vi "Process.vi"(8 "error in":errorcluster, 11 "Inst.Krohn-Hite-7008":refnum<class "Inst.Krohn-Hite-7008.lvclass">) -> (0 "error out":errorcluster, 3 "Inst.Krohn-Hite-7008 out":refnum<class "Inst.Krohn-Hite-7008.lvclass">)   [LabVIEW 2019, in "Inst.KH7008.lvlib" / "Inst.Krohn-Hite-7008.lvclass"]
doc: "---------------------------------------------------------------\nJKI State Machine Objects™\nhttp://jki.net/state-machine-objects/\nCopyright (C) 2005-2015, JKI <info@jki.net>\nALL RIGHTS RESERVED"
uses:
  Inst.Krohn-Hite-7008.lvclass
  <userlib>/LevyLab/Instrument Framework/Instrument/Instrument.lvclass
  <userlib>/LevyLab/RemoteControl/RemoteControl/Typedefs/Message--Cluster.ctl
  <userlib>/LevyLab/RemoteControl/RemoteControl/RemoteControl.lvclass
  Typedefs/PrivateEvents--Inst.KH7008.MessageToProcess.ctl
  Typedefs/Inst.KH7008.Commands--Enum.ctl
  Typedefs/Inst.KH7008.ProtectedCommands--Enum.ctl
  KH7008/KH7008.lvlib
  ef847fcc-ae38-4c9a-a9d7-f0d56e5c7fa0.vi
  <userlib>/LevyLab/Debug/Debug.lvlib
  KH7008/typedefs/channel--numeric.ctl
  KH7008/typedefs/gain--enum.ctl
  KH7008/typedefs/Input--Enum.ctl
  KH7008/typedefs/shunt--enum.ctl
  KH7008/typedefs/couple--Enum.ctl
  KH7008/typedefs/Filter--Enum.ctl
  KH7008/typedefs/channelProperties--Cluster.ctl
  KH7008/typedefs/allChannelProperties--Array.ctl
  Typedefs/getAllChannelsResponse--Cluster.ctl
  Typedefs/getAllChannelsDatabase--Cluster.ctl
  Typedefs/Inst.KH7008.getAll--Cluster.ctl
  Typedefs/setAllChannelsRequest--Cluster.ctl
  Typedefs/PublicEvents--Inst.KH7008.MessageFromProcess.ctl
  Typedefs/PublicEvents--Cluster.ctl
  <vilib>/JKI/JKI SMO/SMO/SMO.lvclass
  <userlib>/LevyLab/Instrument Framework/Instrument Types/Amplifier/Instrument.Amplifier.lvclass
  c2686cc3-20e9-4710-a87a-2e2b9cb24138.vi
  0289f19f-f572-4acd-b603-fc7faa2e8eca.vi
  <userlib>/LevyLab/Instrument Framework/Instrument/API/Instrument.sendMessageToProcess (variant).vi
  C:/Program Files/National Instruments/LabVIEW 2019/user.lib/LevyLab/Instrument Framework/Instrument Types/Amplifier/Instrument.Amplifier.lvclass
  C:/Program Files/National Instruments/LabVIEW 2019/user.lib/LevyLab/Instrument Framework/Instrument/Instrument.lvclass
  C:/Program Files/National Instruments/LabVIEW 2019/vi.lib/JKI/JKI SMO/SMO/SMO.lvclass
panel:
  out "device":string
  out "Status":string
  out "State History":string
  # "Krohn-Hite-7008"
  # "Instrument.Krohn-Hite-7008"
  # "For instructions on how to use the JKI State Machine Objects, examples and video tutorials, visit:\nhttp://jki.net/state-machine-objects/\n\nJKI State Machine Objects™\nhttp://jki.net/state-machine-objects/\nCopyright (C) 2005-2015, JKI <info@jki.net>\nALL RIGHTS RESERVED"
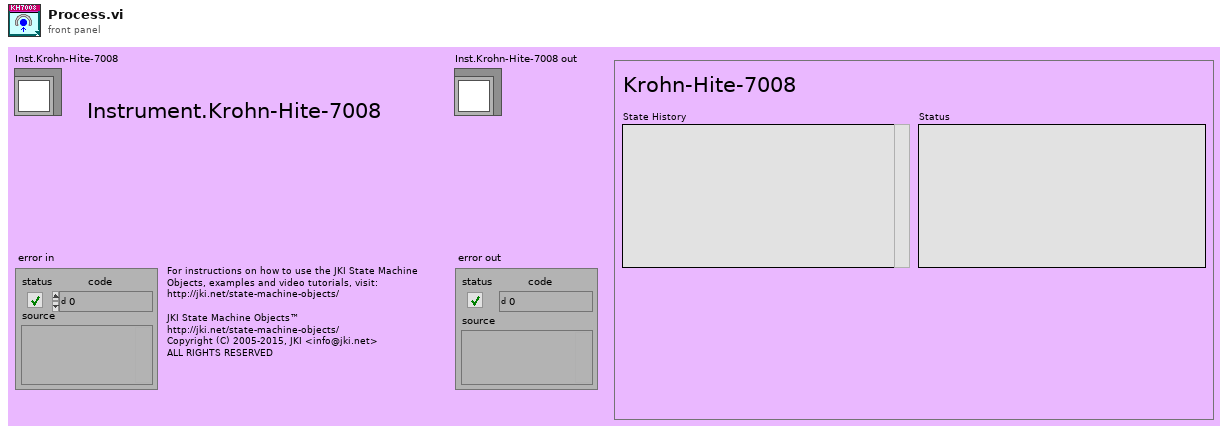
[diagram p1: front panel]
types:
  T1 = typedef "Inst.KH7008.lvlib/Inst.Krohn-Hite-7008.lvclass/Inst.KH7008.Commands--Enum.ctl" = enum16{"getChannel", "getAllChannels", "setChannel", "setAllChannels", "getShuntResistor", "getChassis"}
  T2 = typedef "Inst.KH7008.lvlib/Inst.Krohn-Hite-7008.lvclass/Inst.KH7008.getAll--Cluster.ctl" = cluster{"allChannelProperties":T3}
  T3 = typedef "KH7008.lvlib/allChannelProperties--Array.ctl" = T4[]
  T4 = typedef "KH7008.lvlib/channelProperties--Cluster.ctl" = cluster{"channel":T5, "gain":T6, "input":T7, "shunt":T8, "couple":T9, "filter":T10}
  T5 = typedef "KH7008.lvlib/channel--numeric.ctl" = u16
  T6 = typedef "KH7008.lvlib/gain--enum.ctl" = enum16{"1", "10", "100", "1000"}
  T7 = typedef "KH7008.lvlib/Input--Enum.ctl" = enum16{"OFF", "SE+", "SE-", "DIFF"}
  T8 = typedef "KH7008.lvlib/shunt--enum.ctl" = enum16{"Open", "50", "500", "5k", "50k", "10M"}
  T9 = typedef "KH7008.lvlib/couple--Enum.ctl" = enum16{"AC", "DC"}
  T10 = typedef "KH7008.lvlib/Filter--Enum.ctl" = enum16{"OFF", "ON"}
  T11 = typedef "Inst.KH7008.lvlib/Inst.Krohn-Hite-7008.lvclass/PublicEvents--Cluster.ctl" = cluster{"MessageFromProcess":refnum<user-event>}
  T12 = cluster{"VISA resource":refnum<visa-resource-name>, "getAll":T2, "Private Events":cluster{"MessageToProcess":refnum<user-event>}, "Public Events":T11}
  T13 = typedef "Inst.KH7008.lvlib/Inst.Krohn-Hite-7008.lvclass/setAllChannelsRequest--Cluster.ctl" = cluster{"allChannelProperties":T3}
  T14 = typedef "Inst.KH7008.lvlib/Inst.Krohn-Hite-7008.lvclass/getAllChannelsDatabase--Cluster.ctl" = cluster{"channel":u32, "gain":string, "input":string, "shunt":string, "couple":string, "filter":string, "model":string, "device_id":string}
  T15 = typedef "Inst.KH7008.lvlib/Inst.Krohn-Hite-7008.lvclass/getAllChannelsResponse--Cluster.ctl" = cluster{"allChannelProperties":T3}
  T16 = enum32{"invalid app kind", "Development System", "Run Time System", "Student Edition", "Embedded LabVIEW", "Evaluation", "Custom"}
  T17 = enum32{"Invalid", "Standard", "Closed", "Hidden", "Minimized", "Maximized"}
  T18 = typedef "Inst.KH7008.lvlib/Inst.Krohn-Hite-7008.lvclass/Inst.KH7008.ProtectedCommands--Enum.ctl" = enum16{"setAllChannelProperties", "setSR"}
  T19 = typedef "Inst.KH7008.lvlib/Inst.Krohn-Hite-7008.lvclass/PrivateEvents--Inst.KH7008.MessageToProcess.ctl" = cluster{"Message":T20}
  T20 = typedef "RemoteControl.lvlib/RemoteControl.lvclass/Message--Cluster.ctl" = cluster{"Command":string, "Data":variant, "ID":string, "error":errorcluster}
  T21 = cluster{"Core":cluster{"Current VI Reference":refnum<vi>, "Close Panel on Exit?":bool, "Last Error":cluster{"error":errorcluster, "previous state":string, "remaining states":string}, "Shutdown?":bool}, "SMO":refnum<class "Inst.Krohn-Hite-7008.lvclass">, "Running Step":i32, "sequence":string[], "MessageToProcess":T19}
  T22 = cluster{"Current VI Reference":refnum<vi>, "Close Panel on Exit?":bool, "Last Error":cluster{"error":errorcluster, "previous state":string, "remaining states":string}, "Shutdown?":bool}
  T23 = typedef "Debug.lvlib/Attribute.Debug.lvclass/DebugBehavior.ctl" = enum16{"Normal", "Debug"}
  T24 = typedef "SMO.lvclass/Protected Events.ctl" = cluster{"StopProcesses":refnum<user-event>, "AbortProcesses":refnum<user-event>, "Config Changed":refnum<user-event>, "Dependency":refnum<user-event>}
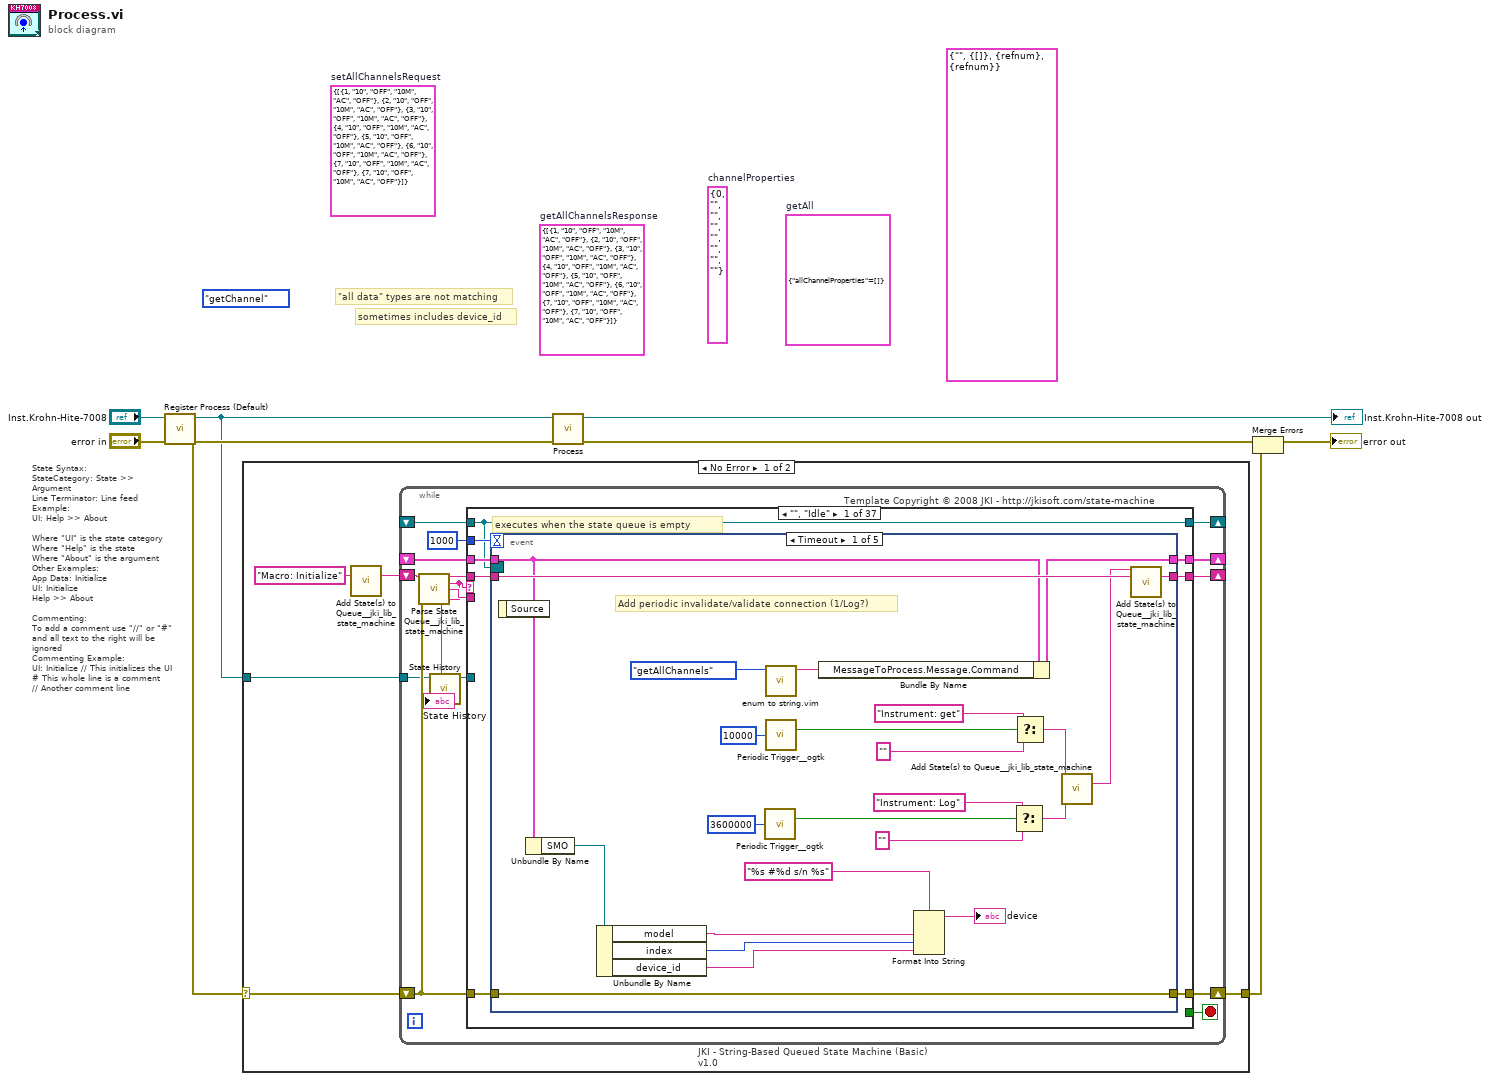
[diagram p0: block diagram]
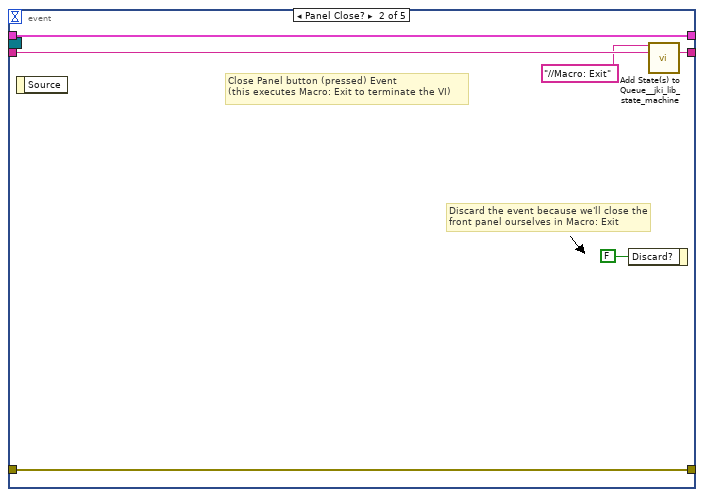
[diagram p2: hidden frame]
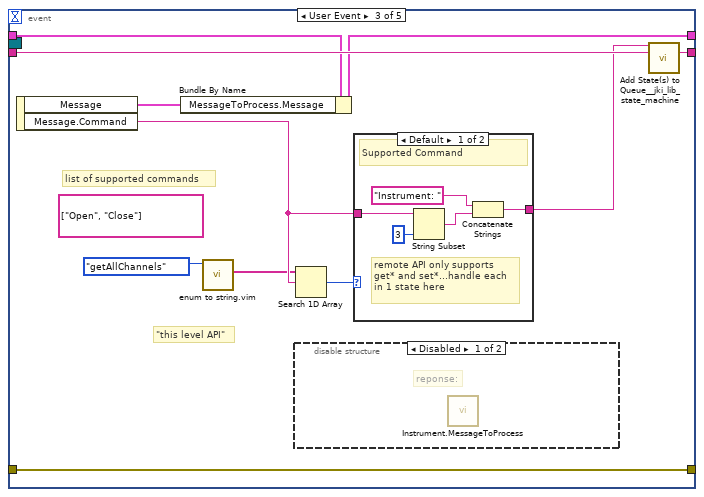
[diagram p3: hidden frame]
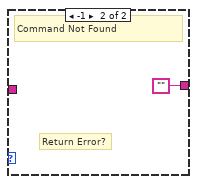
[diagram p5: hidden frame]
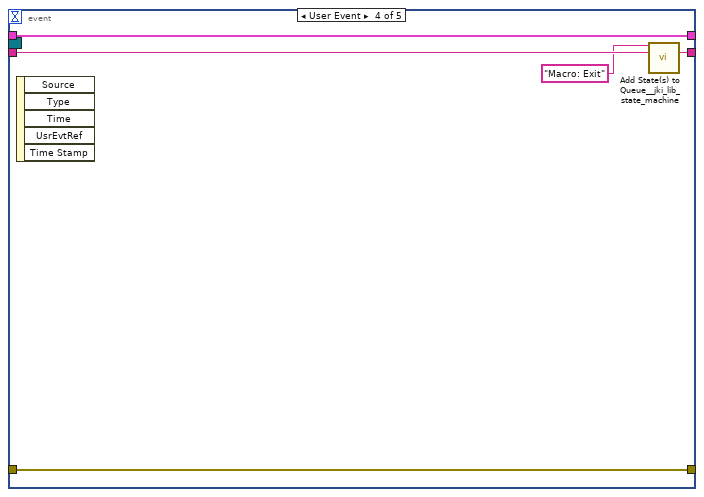
[diagram p6: hidden frame]
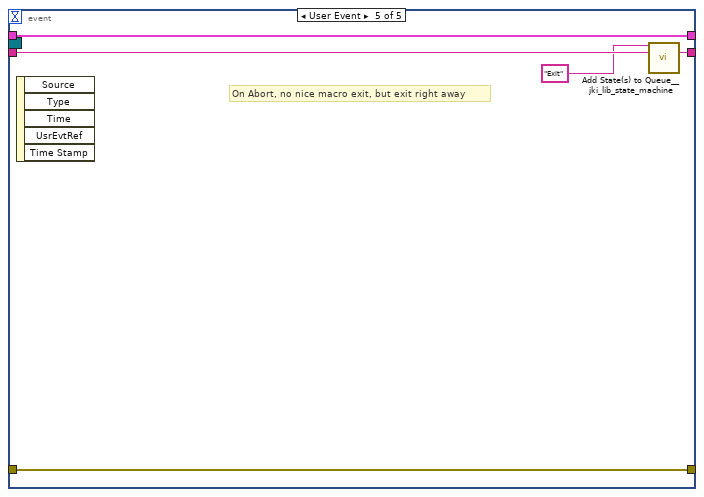
[diagram p7: hidden frame]
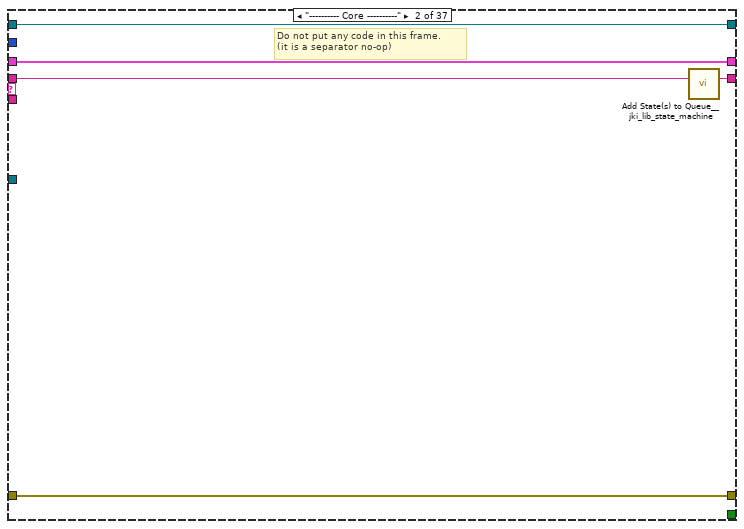
[diagram p8: hidden frame]
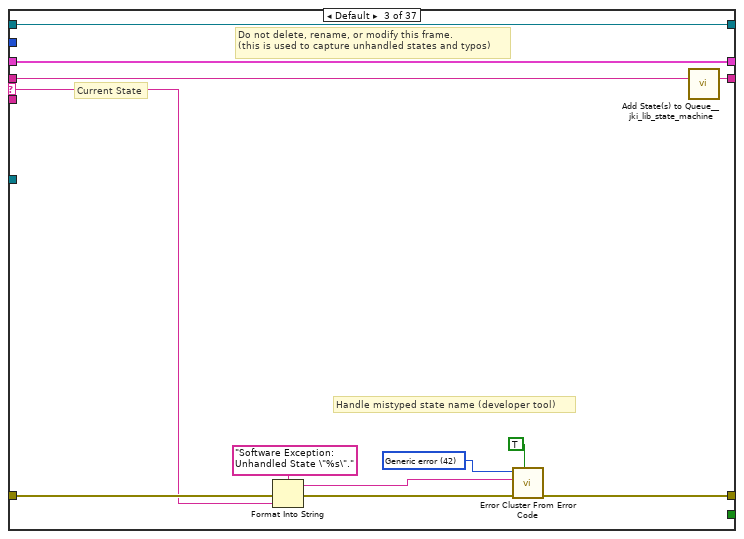
[diagram p9: hidden frame]
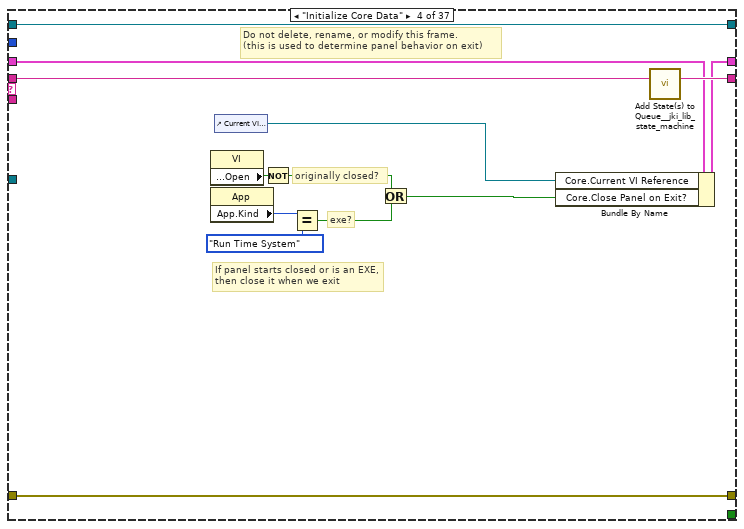
[diagram p10: hidden frame]
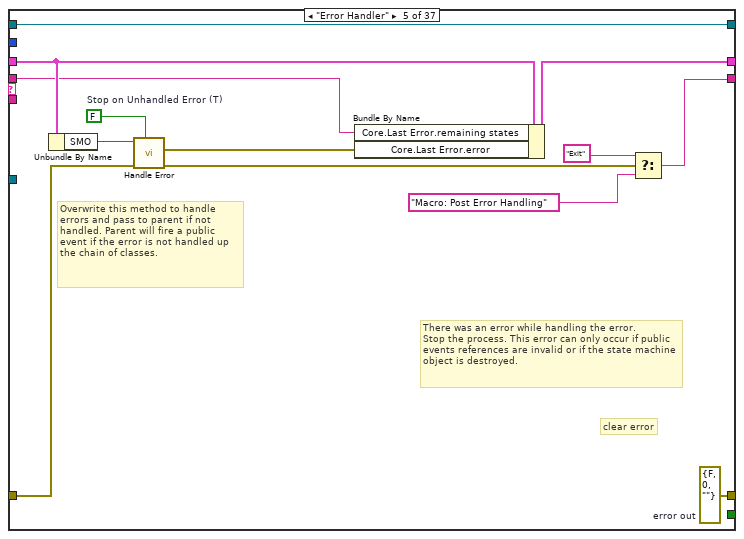
[diagram p11: hidden frame]
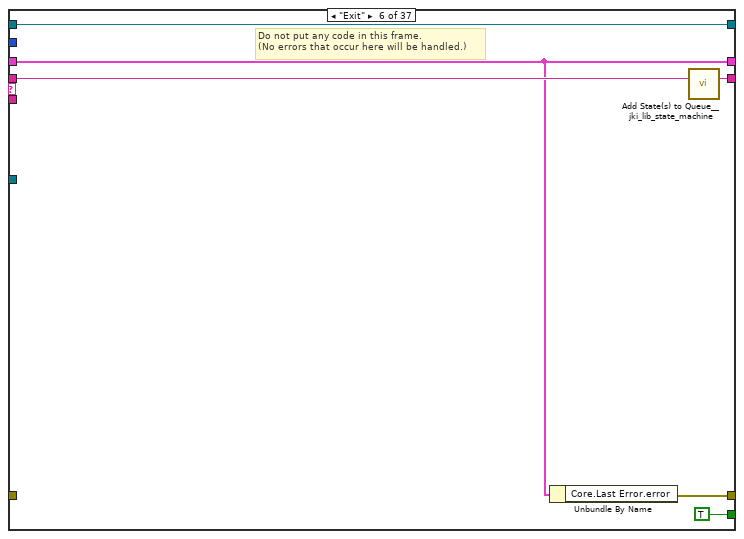
[diagram p12: hidden frame]
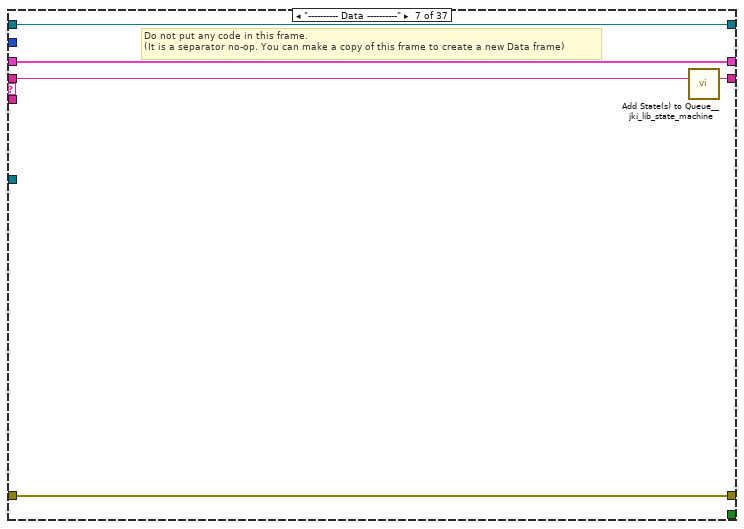
[diagram p13: hidden frame]
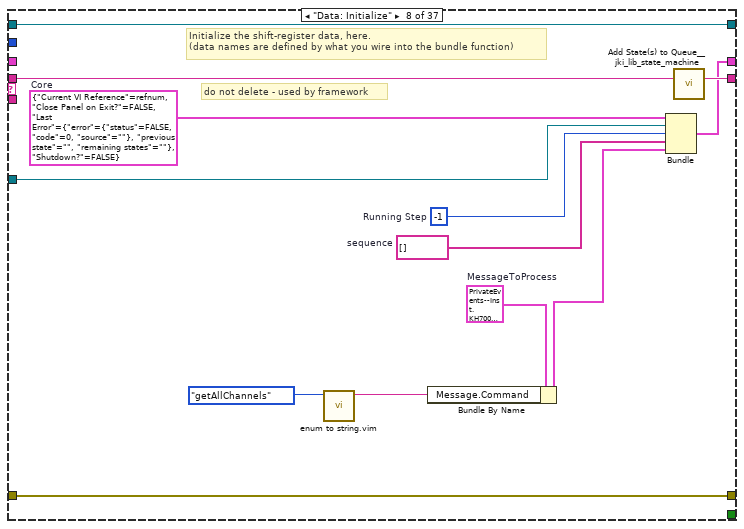
[diagram p14: hidden frame]
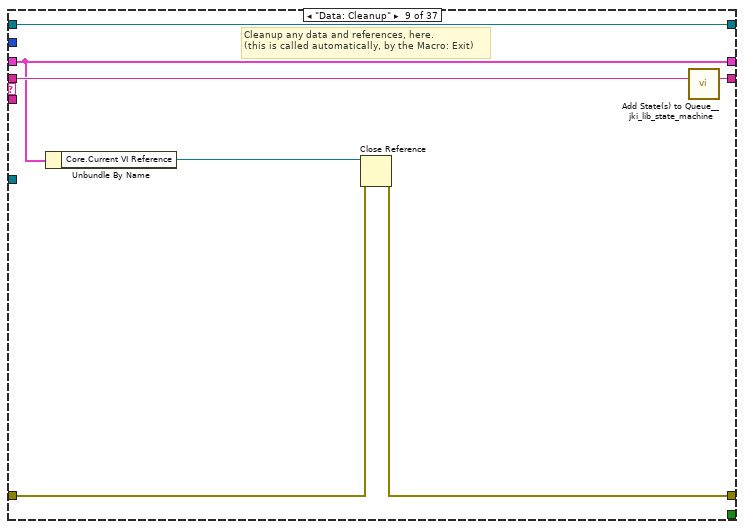
[diagram p15: hidden frame]
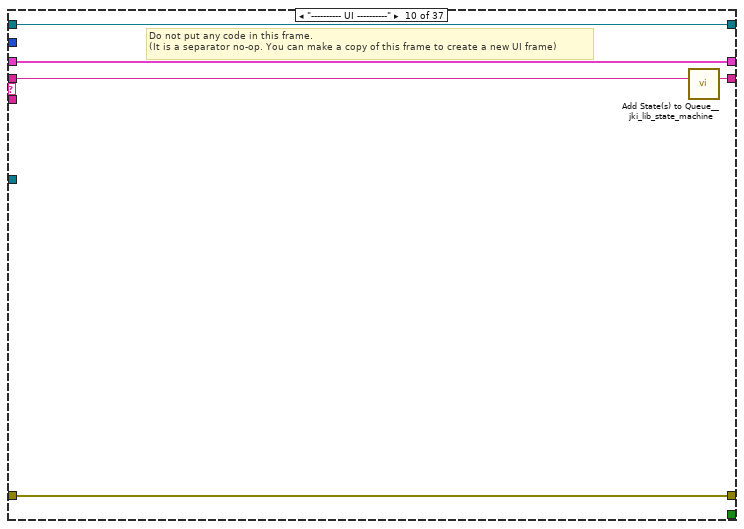
[diagram p16: hidden frame]
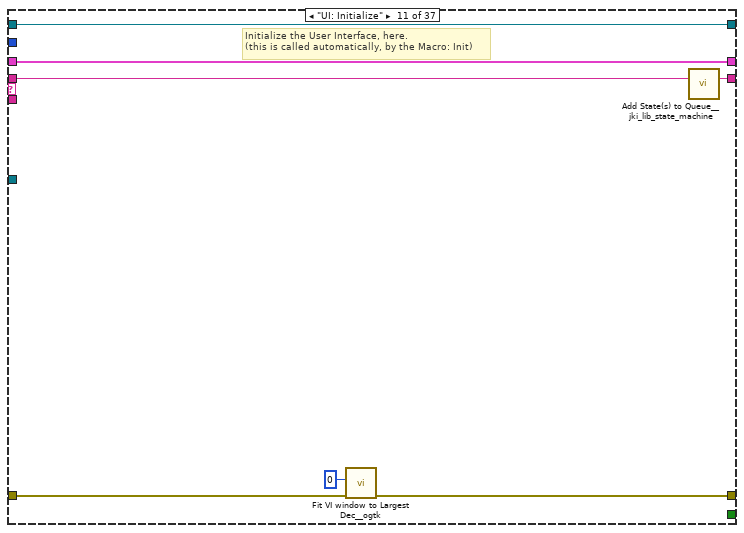
[diagram p17: hidden frame]
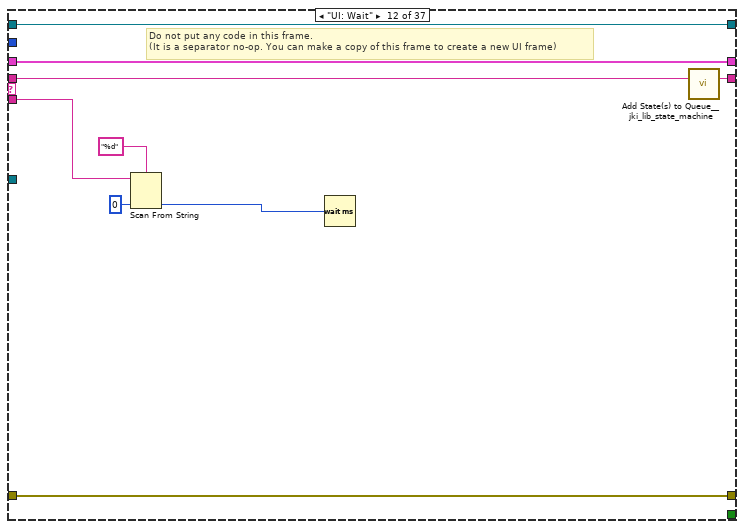
[diagram p18: hidden frame]
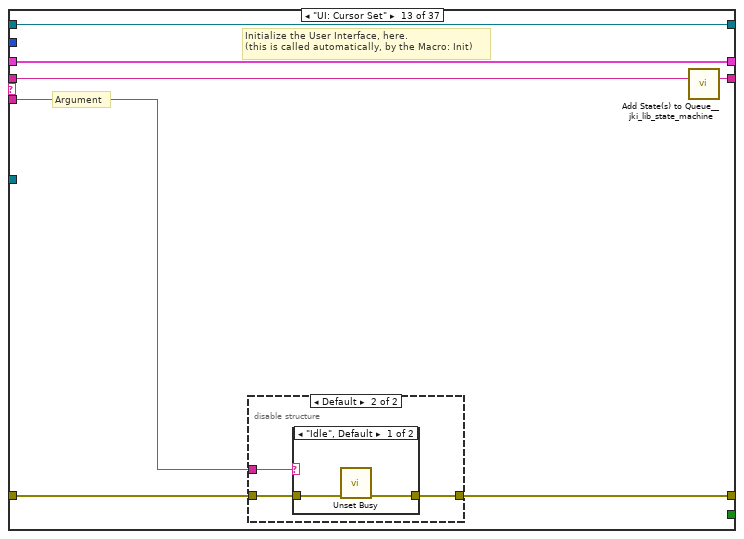
[diagram p19: hidden frame]
diagram:
  (unwired) Inst.KH7008.Commands--Enum."getChannel" ("publicCommands")
  (unwired) T12 {"VISA resource"="", "getAll"={"allChannelProperties"=[]}, "Private Events"={"MessageToProcess"=refnum}, "Public Events"={"MessageFromProcess"=refnum}} ("Cluster of class private data")
  (unwired) T13 {"allChannelProperties"=[{"channel"=1, "gain"=enum."10", "input"=enum."OFF", "shunt"=enum."10M", "couple"=enum."AC", "filter"=enum."OFF"}, {"channel"=2, "gain"=enum."10", "input"=enum."OFF", "shunt"=enum."10M", "couple"=enum."AC", "filter"=enum."OFF"}, {"channel"=3, "gain"=enum."10", "input"=enum."OFF", "shunt"=enum."10M", "couple"=enum."AC", "filter"=enum."OFF"}, {"channel"=4, "gain"=enum."10", "input"=enum."OFF", "shunt"=enum."10M", "couple"=enum."AC", "filter"=enum."OFF"}, {"channel"=5, "gain"=enum."10", "input"=enum."OFF", "shunt"=enum."10M", "couple"=enum."AC", "filter"=enum."OFF"}, {"channel"=6, "gain"=enum."10", "input"=enum."OFF", "shunt"=enum."10M", "couple"=enum."AC", "filter"=enum."OFF"}, {"channel"=7, "gain"=enum."10", "input"=enum."OFF", "shunt"=enum."10M", "couple"=enum."AC", "filter"=enum."OFF"}, {"channel"=7, "gain"=enum."10", "input"=enum."OFF", "shunt"=enum."10M", "couple"=enum."AC", "filter"=enum."OFF"}]}  # setAllChannelsRequest
  (unwired) T2 {"allChannelProperties"=[]}  # getAll
  (unwired) T14 {"channel"=0, "gain"="", "input"="", "shunt"="", "couple"="", "filter"="", "model"="", "device_id"=""}  # channelProperties
  (unwired) T15 {"allChannelProperties"=[{"channel"=1, "gain"=enum."10", "input"=enum."OFF", "shunt"=enum."10M", "couple"=enum."AC", "filter"=enum."OFF"}, {"channel"=2, "gain"=enum."10", "input"=enum."OFF", "shunt"=enum."10M", "couple"=enum."AC", "filter"=enum."OFF"}, {"channel"=3, "gain"=enum."10", "input"=enum."OFF", "shunt"=enum."10M", "couple"=enum."AC", "filter"=enum."OFF"}, {"channel"=4, "gain"=enum."10", "input"=enum."OFF", "shunt"=enum."10M", "couple"=enum."AC", "filter"=enum."OFF"}, {"channel"=5, "gain"=enum."10", "input"=enum."OFF", "shunt"=enum."10M", "couple"=enum."AC", "filter"=enum."OFF"}, {"channel"=6, "gain"=enum."10", "input"=enum."OFF", "shunt"=enum."10M", "couple"=enum."AC", "filter"=enum."OFF"}, {"channel"=7, "gain"=enum."10", "input"=enum."OFF", "shunt"=enum."10M", "couple"=enum."AC", "filter"=enum."OFF"}, {"channel"=7, "gain"=enum."10", "input"=enum."OFF", "shunt"=enum."10M", "couple"=enum."AC", "filter"=enum."OFF"}]}  # getAllChannelsResponse
  # "sometimes includes device_id"
  # "\"all data\" types are not matching"
  # "State Syntax:\nStateCategory: State >> Argument\nLine Terminator: Line feed\nExample:\nUI: Help >> About\n\nWhere \"UI\" is the state category\nWhere \"Help\" is the state\nWhere \"About\" is the argument\nOther Examples:\nApp Data: Initialize\nUI: Initialize\nHelp >> About\n\nCommenting:\nTo add a comment use \"//\" or \"#\" and all text to the right will be ignored\nCommenting Example:\nUI: Initialize // This initializes the UI\n# This whole line is a comment\n// Another comment line"
  n1 = call <vilib>:"Register Process (Default).vi"("error in (no error)"="error in", "SMO"="Inst.Krohn-Hite-7008") -> ("error out"=w5:errorcluster, "SelfRef"=w4:refnum<class "Inst.Krohn-Hite-7008.lvclass">)  [unwired: 8 in]
  n2 = case shown="No Error" w5 {
    selector: w5 -> [w10 w532]
    tunnel: w4 -> [w11 _]
    tunnel: [w9 w532] -> w1
    frame No Error {
      n3 = call <vilib>:"Add State(s) to Queue__jki_lib_state_machine.vi"("State(s) in (\"\")"="Macro: Initialize") -> ("States Out"=w13:string)  [unwired: 14 in]
      n4 = while "JKI - String-Based Queued State Machine (Basic) v1.0" {
        shift-right: [w23] -> _
        shift-left: _ -> [w22]
        shift-right: [w26] -> w9
        shift-left: w10 -> [w20]
        shift-right: [w25] -> _
        shift-left: w13 -> [w27]
        tunnel: w11 -> [w14]
        shift-right: [w19] -> _
        shift-left: _ -> [w18]
        stop <- w24 stop-if-true
        # "Template Copyright © 2008 JKI - http://jkisoft.com/state-machine"
        n5 = call <vilib>:"Parse State Queue__jki_lib_state_machine.vi"("State Queue"=w27, "Error In (no error)"=w20) -> ("Remaining States"=w29:string, "Current State"=w17:string, "Arguments"=w28:string)  [unwired: 11 in]
        n6 = call <userlib>:"State History.vi"("Current State"=w17, "SMO"=w14) -> ("SMO"=w15:refnum<class "Inst.Krohn-Hite-7008.lvclass">, "History"=→"State History":string)  [unwired: 8 in]
        n7 = case shown="\"\", \"Idle\"" w17 {
          selector: w17 -> [_ _ w101 _ _ _ _ _ _ _ _ _ _ _ _ _ _ _ _ _ _ _ _ _ _ _ _ _ _ _ _ _ _ _ _ _ _]
          tunnel: w29 -> [w37 w99 w105 w124 w129 w143 w148 w161 w168 w173 w180 w189 w196 w212 w244 w253 w268 w280 _ w323 w340 w345 w356 w363 w368 w381 w387 w394 w403 w418 w438 w466 w485 w501 w506 w512 w531]
          tunnel: w28 -> [_ _ _ _ _ _ _ _ _ _ _ w181 w190 w206 _ _ _ _ _ _ _ _ _ _ _ _ _ _ _ _ _ _ _ _ _ w507 w515]
          tunnel: w22 -> [w35 w96 w103 w115 w133 w139 w145 _ w163 w170 w178 w186 w194 w208 w241 w250 w257 w277 w283 w313 w324 w342 w353 w360 w365 w374 w385 w389 w399 w414 w434 w462 w481 w497 w502 w508 w521]
          tunnel: [w34 w97 w107 w121 w134 w138 w146 w153 w164 w171 w175 w187 w191 w209 w242 w245 w255 w278 w291 w321 w327 w343 w347 w358 w366 w377 w383 w391 w395 w404 w431 w458 w470 w494 w503 w509 w523] -> w26
          tunnel: w20 -> [w33 w97 w106 w121 w135 _ w146 w153 w165 w171 w174 w187 w192 w210 w242 w245 w254 w278 w291 w321 w327 w343 w348 w357 w366 w371 w383 w391 w397 w412 w430 w459 w473 w493 w503 w509 w517]
          tunnel: [w36 w98 w104 w123 w125 w142 w147 w160 w167 w172 w179 w188 w195 w211 w243 w252 w267 w279 w292 w322 w339 w344 w355 w362 w367 w380 w386 w393 w402 w417 w437 w465 w484 w500 w505 w511 w530] -> w25
          tunnel: [_ _ _ _ _ TRUE _ _ _ _ _ _ _ _ _ _ _ _ _ _ _ _ _ _ _ _ _ _ _ _ _ _ _ _ _ _ _] -> w24
          tunnel: [w32 w96 w103 w122 w132 w139 w145 w159 w163 w170 w178 w186 w194 w208 w241 w250 w258 w277 w284 w314 w325 w342 w353 w360 w365 w374 w385 w390 w400 w415 w435 w463 w482 w498 w502 w508 w520] -> w23
          tunnel: 1000 ("Timeout") -> [w31 _ _ _ _ _ _ _ _ _ _ _ _ _ _ _ _ _ _ _ _ _ _ _ _ _ _ _ _ _ _ _ _ _ _ _ _]
          tunnel: w15 -> [_ _ _ _ _ _ _ w154 _ _ _ _ _ _ _ _ _ _ _ _ _ _ _ _ _ _ _ _ _ _ _ _ _ _ _ _ _]
          tunnel: [w30 w95 w100 w112 w137 w140 w144 w158 w162 w169 w177 w185 w193 w205 w240 w251 w266 w276 w290 w320 w335 w341 w354 w361 w364 w379 w384 w392 w401 w416 w436 w464 w483 w499 w504 w510 w529] -> w19
          tunnel: w18 -> [w30 w95 w100 w112 w137 w140 w144 w158 w162 w169 w177 w185 w193 w205 w240 w251 w266 w276 w290 w320 w335 w341 w354 w361 w364 _ w384 w392 w401 w416 w436 w464 w483 w499 w504 w510 w529]
          frame "", "Idle" {
            # "executes when the state queue is empty"
            n8 = event shown="[0] Timeout" {
              selector: w30 -> [_ _ _ _ _]
              dyn-events: _ -> [_ _ _ _ _]
              timeout: w31 -> [_ _ _ _ _]
              tunnel: w37 -> [w61 w67 w78 w89 w94]
              tunnel: [w60 w66 w77 w88 w93] -> w36
              tunnel: w35 -> [w42 w64 w71 w86 w91]
              tunnel: [w59 w65 w76 w87 w92] -> w34
              tunnel: w33 -> [w59 w65 w76 w87 w92]
              tunnel: [w56 w64 w72 w86 w91] -> w32
              event Timeout {
                # "Add periodic invalidate/validate connection (1/Log?)"
                n9 = event-data() -> ()  [unwired: 1 in, 1 out]
                n10 = Unbundle By Name(w42) -> ("SMO"=w41:refnum<class "Inst.Krohn-Hite-7008.lvclass">)
                n11 = Unbundle By Name(w41) -> ("model"=w40:string, "index"=w39:i32, "device_id"=w38:string)
                n12 = call <userlib>:"Periodic Trigger__ogtk.vi"("time (ms)"=u32 3600000) -> ("Triggered"=w48:bool)  [unwired: 12 in, 2 out]
                n13 = call "enum to string.vim"("enum in"=Inst.KH7008.Commands--Enum."getAllChannels" ("Commands")) -> ("string out"=w58:string)  [unwired: 9 in, 1 out]
                n14 = call <userlib>:"Periodic Trigger__ogtk.vi"("time (ms)"=u32 10000) -> ("Triggered"=w55:bool)  [unwired: 12 in, 2 out]
                n15 = Bundle By Name(cluster=w42, "MessageToProcess.Message.Command"=w58) -> (w56:T21)
                n16 = Format Into String(format string="%s #%d s/n %s", w40, w39, w38) -> (resulting string=→"device":string)  [unwired: 2 in, 1 out]
                n17 = Select(t="Instrument: Log", s=w48, f="") -> (s? t:f=w47:string)
                n18 = Select(t="Instrument: get", s=w55, f="") -> (s? t:f=w46:string)
                n19 = call <vilib>:"Add State(s) to Queue__jki_lib_state_machine.vi"("State(s) in Front (\"\")"=w46, "State(s) at Back (\"\")"=w47) -> ("States Out"=w45:string)  [unwired: 13 in]
                n20 = call <vilib>:"Add State(s) to Queue__jki_lib_state_machine.vi"("State(s) in Front (\"\")"=w45, "State(s) in (\"\")"=w61) -> ("States Out"=w60:string)  [unwired: 13 in]
              }
              event Panel Close? {
                # "Discard the event because we'll close the front panel ourselves in Macro: Exit"
                # "Close Panel button (pressed) Event\n(this executes Macro: Exit to terminate the VI)"
                n21 = event-data() -> ()  [unwired: 1 in, 1 out]
                n22 = event-data("Discard?"=FALSE) -> ()  [unwired: 1 in, 1 out]
                n23 = call <vilib>:"Add State(s) to Queue__jki_lib_state_machine.vi"("State(s) in Front (\"\")"="//Macro: Exit", "State(s) in (\"\")"=w67) -> ("States Out"=w66:string)  [unwired: 13 in]
              }
              event User Event {
                (unwired) string[] ["Open", "Close"]
                # "\"this level API\""
                # "list of supported commands"
                n24 = event-data() -> ("Message"=w70:T20, "Message.Command"=w73:string)  [unwired: 1 in]
                n25 = Bundle By Name(cluster=w71, "MessageToProcess.Message"=w70) -> (w72:T21)
                n26 = call "enum to string.vim"("enum in"=Inst.KH7008.Commands--Enum."getAllChannels" ("Commands")) -> ("strings out"=w68:string[])  [unwired: 9 in, 1 out]
                n27 = disable-structure shown="Disabled" {
                  frame Disabled {
                    # "reponse:"
                    n28 = call <userlib>:"Instrument.MessageToProcess.vi"() -> ()  [unwired: 10 in, 2 out]
                  }
                  frame Enabled {
                  }
                }
                n29 = Search 1D Array(1D array=w68, element=w73) -> (index of element=w75:i32)  [unwired: 1 in]
                n30 = case shown="Default" w75 {
                  tunnel: [w83 "" ("Empty String Constant")] -> w74
                  tunnel: w73 -> [w79 _]
                  frame Default {
                    # "remote API only supports\nget* and set*...handle each \nin 1 state here"
                    # "Supported Command"
                    n31 = String Subset(string=w79, length (rest)=3 ("length (rest)")) -> (substring=w80:string)  [unwired: 1 in]
                    n32 = Concatenate Strings("Instrument: ", w80) -> (w83:string)
                  }
                  frame -1 {
                    # "Return Error?"
                    # "Command Not Found"
                  }
                }
                n33 = call <vilib>:"Add State(s) to Queue__jki_lib_state_machine.vi"("State(s) in Front (\"\")"=w74, "State(s) in (\"\")"=w78) -> ("States Out"=w77:string)  [unwired: 13 in]
              }
              event User Event {
                n34 = event-data() -> ()  [unwired: 1 in, 5 out]
                n35 = call <vilib>:"Add State(s) to Queue__jki_lib_state_machine.vi"("State(s) in Front (\"\")"="Macro: Exit", "State(s) in (\"\")"=w89) -> ("States Out"=w88:string)  [unwired: 13 in]
              }
              event User Event {
                # "On Abort, no nice macro exit, but exit right away"
                n36 = event-data() -> ()  [unwired: 1 in, 5 out]
                n37 = call <vilib>:"Add State(s) to Queue__jki_lib_state_machine.vi"("State(s) in Front (\"\")"="Exit", "State(s) in (\"\")"=w94) -> ("States Out"=w93:string)  [unwired: 13 in]
              }
            }
          }
          frame "---------- Core ----------" {
            # "Do not put any code in this frame.\n(it is a separator no-op)"
            n38 = call <vilib>:"Add State(s) to Queue__jki_lib_state_machine.vi"("State(s) in (\"\")"=w99) -> ("States Out"=w98:string)  [unwired: 14 in]
          }
          frame Default {
            w110 = 42 items=["No error", "Argument error", "Memory is full", "Out of zone", "End of file", "File already open", "Generic file I/O error", "File not found", "File permission error", "Disk is full", "Duplicate path", "Too many files open", "System feature not enabled", "Resource file not found", "Cannot add resource", "Resource not found", "Image not found", "Image memory error", "Pen does not exist", "Config type invalid", "Config token not found", "Config parse error", "Config memory error", "Bad external code format", "Bad external code offset", "External code not present", "Null window", "Destroy window error", "Null menu", "Print aborted", "Bad print record", "Print driver error", "Windows error during printing", "Memory error during printing", "Print dialog error", "Generic print error", "Invalid device refnum", "Device not found", "Device parameter error", "Device unit error", "Cannot open device", "Device call aborted", "Generic error", "Cancelled by user", "Object ID too low", "Object ID too high", "Object not in heap", "Unknown heap", "Unknown object (invalid DefProc)", "Unknown object (DefProc not in table)", "Message out of range", "Invalid (null) method", "Unknown message", "Manager call not supported", "Bad address", "Network operation in progress", "Network operation timed out", "Connection is busy", "Network attribute not supported", "Network error", "Address in use", "System out of memory", "Connection aborted", "Connection refused", "Not connected", "Already connected", "Connection closed", "Initialization error (interapplication manager)", "Bad occurrence", "Wait on unbound occurrence handler", "Occurrence queue overflow", "Datalog type conflict", "Unused", "Unrecognized type (interapplication manager)", "Memory corrupt", "Failed to make temporary DLL", "Old CIN version", "Drag socket not found", "Failed to load drop-object", "Failed to register OLE object", "Failed to release OLE object", "Format specifier type mismatch", "Unknown format specifier", "Too few format specifiers", "Too many format specifiers", "Scan failed", "Newer CIN version", "Error converting to variant", "Runtime menu error", "Password tampered", "Variant attribute not found", "Incompatible variant data type", "Event data is not available", "Event Store is not present", "Occurrence is not found", "Event Queue is not created", "Event info is not available", "Refnum passed is NULL", "Error retrieving Class GUID", "Error retrieving CoClass GUID", "Error retrieving TypeLib GUID.", "Bad built application magic bytes.", "Specific driver is different from the specific driver associated with the Logical Name.", "There is no session opened to the class driver.", "Max Error", "MAX - Error with config objects", "MAX - Error loading configuration", "MAX - Group not supported"]
            # "Current State"
            # "Do not delete, rename, or modify this frame.\n(this is used to capture unhandled states and typos)"
            # "Handle mistyped state name (developer tool)"
            n39 = Format Into String(format string="Software Exception: Unhandled State \"%s\"." ("message"), error in=w106, w101) -> (resulting string=w109:string, error out=w108:errorcluster)  [unwired: 1 in]
            n40 = call <vilib>:"Error Cluster From Error Code.vi"("show call chain? (False)"=TRUE, "error in (no error)"=w108, "error message (\"\")"=w109, "error code (0)"=w110) -> ("error out"=w107:errorcluster)  [unwired: 5 in]
            n41 = call <vilib>:"Add State(s) to Queue__jki_lib_state_machine.vi"("State(s) in (\"\")"=w105) -> ("States Out"=w104:string)  [unwired: 14 in]
          }
          frame "Initialize Core Data" {
            # "Do not delete, rename, or modify this frame.\n(this is used to determine panel behavior on exit)"
            # "originally closed?"
            # "exe?"
            # "If panel starts closed or is an EXE, then close it when we exit"
            n42 = property class="VI"() -> ("Front Panel.Open"=w120:bool)  [unwired: 2 in, 2 out]
            n43 = property class="App"() -> ("App.Kind"=w119:T16)  [unwired: 2 in, 2 out]
            n44 = control-ref of="Current VI Reference"() -> (w113:refnum<vi>)
            n45 = Not(x=w120) -> (.not. x?=w117:bool)
            n46 = Equal?(x=w119, y=T16."Run Time System" ("Application:Kind")) -> (x = y?=w116:bool)
            n47 = Or(x=w117, y=w116) -> (x .or. y?=w114:bool)
            n48 = Bundle By Name(cluster=w115, "Core.Current VI Reference"=w113, "Core.Close Panel on Exit?"=w114) -> (w122:T21)
            n49 = call <vilib>:"Add State(s) to Queue__jki_lib_state_machine.vi"("State(s) in (\"\")"=w124) -> ("States Out"=w123:string)  [unwired: 14 in]
          }
          frame "Error Handler" {
            w130 = FALSE  # Stop on Unhandled Error (T)
            w134 = errorcluster {"status"=FALSE, "code"=0, "source"=""}  # error out
            # "clear error"
            # "There was an error while handling the error.\nStop the process. This error can only occur if public events references are invalid or if the state machine object is destroyed."
            # "Overwrite this method to handle errors and pass to parent if not handled. Parent will fire a public event if the error is not handled up the chain of classes."
            n50 = Unbundle By Name(w133) -> ("SMO"=w136:refnum<class "Inst.Krohn-Hite-7008.lvclass">)
            n51 = call-dynamic "Handle Error.vi"("Stop on Unhandled Error (T)"=w130, "error in"=w135, "SMO"=w136) -> ("handling error"=w126:errorcluster, "Unhandled error"=w131:errorcluster)  [unwired: 6 in, 1 out]
            n52 = Bundle By Name(cluster=w133, "Core.Last Error.remaining states"=w129, "Core.Last Error.error"=w131) -> (w132:T21)
            n53 = Select(t="Exit", s=w126, f="Macro: Post Error Handling") -> (s? t:f=w125:string)
          }
          frame "Exit" {
            # "Do not put any code in this frame.\n(No errors that occur here will be handled.)"
            n54 = Unbundle By Name(w139) -> ("Core.Last Error.error"=w138:errorcluster)
            n55 = call <vilib>:"Add State(s) to Queue__jki_lib_state_machine.vi"("State(s) in (\"\")"=w143) -> ("States Out"=w142:string)  [unwired: 14 in]
          }
          frame "---------- Data ----------" {
            # "Do not put any code in this frame.\n(It is a separator no-op. You can make a copy of this frame to create a new Data frame)"
            n56 = call <vilib>:"Add State(s) to Queue__jki_lib_state_machine.vi"("State(s) in (\"\")"=w148) -> ("States Out"=w147:string)  [unwired: 14 in]
          }
          frame "Data: Initialize" {
            w150 = T19 {"Message"={"Command"="", "Data"=variant(string ""), "ID"="", "error"={"status"=FALSE, "code"=0, "source"=""}}}  # MessageToProcess
            w155 = string[] []  # sequence
            w156 = -1  # Running Step
            w157 = T22 {"Current VI Reference"=refnum, "Close Panel on Exit?"=FALSE, "Last Error"={"error"={"status"=FALSE, "code"=0, "source"=""}, "previous state"="", "remaining states"=""}, "Shutdown?"=FALSE}  # Core
            # "do not delete - used by framework"
            # "Initialize the shift-register data, here.\n(data names are defined by what you wire into the bundle function)"
            n57 = call "enum to string.vim"("enum in"=Inst.KH7008.Commands--Enum."getAllChannels" ("Commands")) -> ("string out"=w152:string)  [unwired: 9 in, 1 out]
            n58 = Bundle By Name(cluster=w150, "Message.Command"=w152) -> (w149:T19)
            n59 = Bundle("Core"=w157, "SMO"=w154, "Running Step"=w156, "sequence"=w155, "MessageToProcess"=w149) -> (w159:T21)  [unwired: 1 in]
            n60 = call <vilib>:"Add State(s) to Queue__jki_lib_state_machine.vi"("State(s) in (\"\")"=w161) -> ("States Out"=w160:string)  [unwired: 14 in]
          }
          frame "Data: Cleanup" {
            # "Cleanup any data and references, here.\n(this is called automatically, by the Macro: Exit)"
            n61 = Unbundle By Name(w163) -> ("Core.Current VI Reference"=w166:refnum<vi>)
            n62 = Close Reference(reference=w166, error in (no error)=w165) -> (error out=w164:errorcluster)
            n63 = call <vilib>:"Add State(s) to Queue__jki_lib_state_machine.vi"("State(s) in (\"\")"=w168) -> ("States Out"=w167:string)  [unwired: 14 in]
          }
          frame "---------- UI ----------" {
            # "Do not put any code in this frame.\n(It is a separator no-op. You can make a copy of this frame to create a new UI frame)"
            n64 = call <vilib>:"Add State(s) to Queue__jki_lib_state_machine.vi"("State(s) in (\"\")"=w173) -> ("States Out"=w172:string)  [unwired: 14 in]
          }
          frame "UI: Initialize" {
            # "Initialize the User Interface, here.\n(this is called automatically, by the Macro: Init)"
            n65 = call <userlib>:"Fit VI window to Largest Dec__ogtk.vi"("error in (no error)"=w174, "border spacing (2 px)"=0) -> ("error out"=w175:errorcluster)  [unwired: 4 in, 1 out]
            n66 = call <vilib>:"Add State(s) to Queue__jki_lib_state_machine.vi"("State(s) in (\"\")"=w180) -> ("States Out"=w179:string)  [unwired: 14 in]
          }
          frame "UI: Wait" {
            # "Do not put any code in this frame.\n(It is a separator no-op. You can make a copy of this frame to create a new UI frame)"
            n67 = Scan From String(format string="%d", input string=w181, default 1=u32 0 ("default value 1")) -> (output 1=w182:u32)  [unwired: 2 in, 3 out]
            n68 = Wait (ms)(milliseconds to wait=w182) -> ()  [unwired: 1 out]
            n69 = call <vilib>:"Add State(s) to Queue__jki_lib_state_machine.vi"("State(s) in (\"\")"=w189) -> ("States Out"=w188:string)  [unwired: 14 in]
          }
          frame "UI: Cursor Set" {
            # "Argument"
            # "Initialize the User Interface, here.\n(this is called automatically, by the Macro: Init)"
            n70 = disable-structure shown="Default" {
              disable-tunnel: w192 -> [w197 w200]
              disable-tunnel: [w197 w199] -> w191
              disable-tunnel: w190 -> [_ w198]
              frame condition #0 {
              }
              frame condition #1 (active) {
                n71 = case shown="\"Idle\", Default" w198 {
                  tunnel: w200 -> [w202 w204]
                  tunnel: [w201 w203] -> w199
                  frame "Idle", Default {
                    n72 = call <vilib>:"Unset Busy.vi"("error in (no error)"=w202) -> ("error out"=w201:errorcluster)  [unwired: 10 in]
                  }
                  frame "Busy" {
                    n73 = call <vilib>:"Set Busy.vi"("error in (no error)"=w204) -> ("error out"=w203:errorcluster)  [unwired: 9 in, 1 out]
                  }
                }
              }
            }
            n74 = call <vilib>:"Add State(s) to Queue__jki_lib_state_machine.vi"("State(s) in (\"\")"=w196) -> ("States Out"=w195:string)  [unwired: 14 in]
          }
          frame "UI: Front Panel State" {
            # "Argument"
            # "Set Front Panel Open or Closed\n(Usage: \"UI: Front Panel State >> Open|Close\")"
            n75 = Unbundle By Name(w208) -> ("Core.Current VI Reference"=w207:refnum<vi>)
            n76 = disable-structure shown="TARGET_TYPE==RT" {
              disable-tunnel: w210 -> [w216 w239]
              disable-tunnel: [w215 w239] -> w209
              disable-tunnel: w207 -> [w214 _]
              disable-tunnel: w206 -> [w213 _]
              frame condition #0 (active) {
                n77 = case shown="\"Close\"" w213 {
                  tunnel: w216 -> [w220 w233]
                  tunnel: [w222 w234] -> w215
                  tunnel: w214 -> [w221 w231]
                  frame "Open", Default {
                    n78 = property class="VI"(reference=w221, error in=w220) -> (reference out=w218:refnum<vi>, error out=w219:errorcluster, "FP.State"=w217:T17)
                    n79 = case shown="\"Closed\"" w217 {
                      tunnel: [w225 w228] -> w222
                      tunnel: w219 -> [w224 w228]
                      tunnel: w218 -> [w223 _]
                      frame "Closed" {
                        n80 = invoke class="VI" method="FP.Open"(reference=w223, error in=w224, "Activate"=TRUE, "State"=T17."Standard") -> (error out=w225:errorcluster)  [unwired: 1 in, 4 out]
                      }
                      frame Default {
                      }
                    }
                  }
                  frame "Close" {
                    n81 = property class="VI"(reference=w231, error in=w233) -> (reference out=w230:refnum<vi>, error out=w232:errorcluster, "FP.State"=w229:T17)
                    n82 = case shown="Default" w229 {
                      tunnel: [w235 w238] -> w234
                      tunnel: w232 -> [w235 w237]
                      tunnel: w230 -> [_ w236]
                      frame "Invalid", "Closed" {
                      }
                      frame Default {
                        n83 = invoke class="VI" method="FP.Close"(reference=w236, error in=w237) -> (error out=w238:errorcluster)  [unwired: 1 in, 2 out]
                      }
                    }
                  }
                }
              }
              frame condition #1 {
              }
            }
            n84 = call <vilib>:"Add State(s) to Queue__jki_lib_state_machine.vi"("State(s) in (\"\")"=w212) -> ("States Out"=w211:string)  [unwired: 14 in]
          }
          frame "---------- Macro ----------" {
            # "Do not put any code in this frame.\n(It is a separator no-op. You can make a copy of this frame to create a new Macro frame)"
            n85 = call <vilib>:"Add State(s) to Queue__jki_lib_state_machine.vi"("State(s) in (\"\")"=w244) -> ("States Out"=w243:string)  [unwired: 14 in]
          }
          frame "Macro: Initialize" {
            # "Initialization Macro\n(This is called once, when the VI starts)"
            n86 = call <vilib>:"Add State(s) to Queue__jki_lib_state_machine.vi"("State(s) in Front (\"\")"="Data: Initialize\nInitialize Core Data\nEvents: Register", "State(s) in (\"\")"="Process: Sync", "State(s) at Back (\"\")"="UI: Initialize\nUI: Front Panel State >> Close\nMacro: Debug\nMacro: Initialize KH") -> ("States Out"=w248:string)  [unwired: 12 in]
            n87 = call <vilib>:"Add State(s) to Queue__jki_lib_state_machine.vi"("State(s) in Front (\"\")"=w248, "State(s) in (\"\")"=w253) -> ("States Out"=w252:string)  [unwired: 13 in]
          }
          frame "Macro: Debug" {
            # "exe?"
            # "If pane is an EXE, then close it when we exit"
            # "Macro: Debug\n(get debug behavior, determine UI and determine shutdown behavior)"
            n88 = Unbundle By Name(w257) -> ("Core.Close Panel on Exit?"=w260:bool, "SMO"=w265:refnum<class "Inst.Krohn-Hite-7008.lvclass">)
            n89 = property class="App"() -> ("App.Kind"=w263:T16)  [unwired: 2 in, 2 out]
            n90 = Equal?(x=w263, y=T16."Run Time System" ("Application:Kind")) -> (x = y?=w259:bool)
            n91 = call <userlib>:"Get Debug Mode.vi"("error in (no error)"=w254, "SMO"=w265) -> ("error out"=w255:errorcluster, "Behavior"=w264:T23)  [unwired: 7 in, 1 out]
            n92 = case shown="\"Normal\", Default" w264 {
              tunnel: [w270 w272] -> w261
              tunnel: w260 -> [w270 _]
              tunnel: w259 -> [_ w274]
              tunnel: ["" "UI: Front Panel State >> Open\nUI: Wait >> 1000"] -> w256
              frame "Normal", Default {
                # "respect core.close"
              }
              frame "Debug" {
                # "keep panel open\nunless exe"
                n93 = Or(x=w274, y=FALSE) -> (x .or. y?=w272:bool)
              }
            }
            n94 = Bundle By Name(cluster=w257, "Core.Close Panel on Exit?"=w261) -> (w258:T21)
            n95 = call <vilib>:"Add State(s) to Queue__jki_lib_state_machine.vi"("State(s) in Front (\"\")"=w256, "State(s) in (\"\")"=w268) -> ("States Out"=w267:string)  [unwired: 13 in]
          }
          frame "Macro: Initialize KH" {
            # "Do not put any code in this frame.\n(It is a separator no-op. You can make a copy of this frame to create a new Macro frame)"
            n96 = call <vilib>:"Add State(s) to Queue__jki_lib_state_machine.vi"("State(s) in Front (\"\")"="Instrument: Open Hardware\nInstrument: Get SR\nInstrument: get\nInstrument: Log" ("State(s) in Front (\"\")"), "State(s) in (\"\")"=w280) -> ("States Out"=w279:string)  [unwired: 13 in]
          }
          frame "Macro: Post Error Handling" {
            # "Clear Last Error?"
            n97 = Unbundle By Name(w283) -> ("Core.Last Error.error"=w282:errorcluster, "Core.Last Error.remaining states"=w285:string, "Core.Shutdown?"=w286:bool)
            n98 = Unbundle By Name(w283) -> ("Core.Last Error.error"=w289:errorcluster)
            n99 = case shown="False" FALSE {
              tunnel: w289 -> [w306 _]
              tunnel: [w306 _] -> w288
              frame False {
              }
              frame True {
              }
            }
            n100 = case shown="False" w286 {
              tunnel: w285 -> [w295 w305]
              tunnel: [w294 w304] -> w281
              tunnel: w282 -> [w298 _]
              frame False {
                # "These are the remaining states (at the moment the error occured). States can be altered according to business logic."
                # "NOT SHUTTING DOWN"
                n101 = call <vilib>:"Clear Errors.vi"("error in (no error)"=w298, "specific error code to clear (0: all)"=-9873) -> ("error out"=w293:errorcluster, "specific error cleared?"=w296:bool)  [unwired: 4 in]
                n102 = case shown="True" w296 {
                  tunnel: w295 -> [w299 _]
                  tunnel: [w299 w303] -> w294
                  tunnel: w293 -> [_ _]
                  frame False {
                  }
                  frame True {
                    n103 = call "Device Error Dialog.vi"() -> ("retry?"=w301:bool)  [unwired: 11 in]
                    n104 = Select(t="Macro: Initialize KH", s=w301, f="Macro: Exit") -> (s? t:f=w303:string)
                  }
                }
              }
              frame True {
                # "Developer can decide to alter the states but should be aware that during the shutdown process, there are certain states that must be run for the SMO to properly shut itself (and this process) down. As such, one can add states to perform additional clean-ups, but should append the remaining state to be executed."
                # "SHUTTING DOWN"
                n105 = call <vilib>:"Add State(s) to Queue__jki_lib_state_machine.vi"("State(s) in (\"\")"=w305) -> ("States Out"=w304:string)  [unwired: 14 in]
              }
            }
            n106 = Bundle By Name(cluster=w283, "Core.Last Error.error"=w288) -> (w284:T21)
            n107 = call <vilib>:"Add State(s) to Queue__jki_lib_state_machine.vi"("State(s) in (\"\")"=w281) -> ("States Out"=w292:string)  [unwired: 14 in]
          }
          frame "Macro: Run Sequence" {
            # "0,1,2,3,4,"
            # "5"
            # "Do not put any code in this frame.\n(It is a separator no-op. You can make a copy of this frame to create a new Macro frame)"
            n108 = Unbundle By Name(w313) -> ("sequence"=w309:string[], "Running Step"=w307:i32)
            n109 = Array Size(array=w309) -> (size(s)=w319:i32)
            n110 = Index Array(array=w309, index=w307) -> (element=w308:string)
            n111 = Greater Or Equal?(x=w319, y=w307) -> (x >= y?=w311:bool)
            n112 = Select(t=-1 ("Running Step"), s=w311, f=w307) -> (s? t:f=w318:i32)
            n113 = Bundle By Name(cluster=w313, "Running Step"=w318) -> (w314:T21)
            n114 = Select(t="Sequence: Status >> ...", s=w311, f="Idle //Check Event Structure\nMacro: Run Sequence" ("State(s) at Back (\"\")")) -> (s? t:f=w310:string)
            n115 = call <vilib>:"Add State(s) to Queue__jki_lib_state_machine.vi"("State(s) in Front (\"\")"=w308, "State(s) at Back (\"\")"=w310) -> ("States Out"=w312:string)  [unwired: 13 in]
            n116 = call <vilib>:"Add State(s) to Queue__jki_lib_state_machine.vi"("State(s) in Front (\"\")"=w312, "State(s) in (\"\")"=w323) -> ("States Out"=w322:string)  [unwired: 13 in]
          }
          frame "Macro: Exit" {
            # "Exit Macro\n(This is called once, when the VI exits)"
            n117 = Unbundle By Name(w324) -> ("Core.Close Panel on Exit?"=w329:bool)
            n118 = Bundle By Name(cluster=w324, "Core.Shutdown?"=TRUE) -> (w325:T21)
            n119 = Select(t="UI: Front Panel State >> Close", s=w329, f="" ("Empty String Constant")) -> (s? t:f=w337:string)
            n120 = call <vilib>:"Add State(s) to Queue__jki_lib_state_machine.vi"("State(s) in Front (\"\")"="Data: Cleanup\nEvents: Unregister\nProcess: SelfTerminate", "State(s) in (\"\")"="Process: Sync", "State(s) at Back (\"\")"="Exit") -> ("States Out"=w332:string)  [unwired: 12 in]
            n121 = call <vilib>:"Add State(s) to Queue__jki_lib_state_machine.vi"("State(s) in Front (\"\")"="Instrument: Close Hardware", "State(s) in (\"\")"=w337, "State(s) at Back (\"\")"=w332) -> ("States Out"=w336:string)  [unwired: 12 in]
            n122 = call <vilib>:"Add State(s) to Queue__jki_lib_state_machine.vi"("State(s) in Front (\"\")"=w336, "State(s) in (\"\")"=w340) -> ("States Out"=w339:string)  [unwired: 13 in]
          }
          frame "---------- Process ----------" {
            # "Template Separator\n(You can make a copy of, or modify, this frame)"
            n123 = call <vilib>:"Add State(s) to Queue__jki_lib_state_machine.vi"("State(s) in (\"\")"=w345) -> ("States Out"=w344:string)  [unwired: 14 in]
          }
          frame "Process: Sync" {
            n124 = Unbundle By Name(w353) -> ("SMO"=w349:refnum<class "Inst.Krohn-Hite-7008.lvclass">)
            n125 = call <vilib>:"WaitOnProcessSync.vi"("error in (no error)"=w348, "SMO"=w349) -> ("error out"=w347:errorcluster, "Don't run?"=w352:bool)  [unwired: 7 in, 1 out]
            n126 = Select(t="Data: Cleanup\nEvents: Unregister\nExit", s=w352, f="" ("Empty String Constant")) -> (s? t:f=w346:string)
            n127 = call <vilib>:"Add State(s) to Queue__jki_lib_state_machine.vi"("State(s) in Front (\"\")"=w346, "State(s) in (\"\")"=w356) -> ("States Out"=w355:string)  [unwired: 13 in]
          }
          frame "Process: SelfTerminate" {
            # "Process: SelfTerminate\n(You can make a copy of, or modify, this frame)"
            n128 = Unbundle By Name(w360) -> ("SMO"=w359:refnum<class "Inst.Krohn-Hite-7008.lvclass">)
            n129 = call <vilib>:"SelfTerminate.vi"("error in (no error)"=w357, "SMO in"=w359) -> ("error out"=w358:errorcluster)  [unwired: 8 in, 1 out]
            n130 = call <vilib>:"Add State(s) to Queue__jki_lib_state_machine.vi"("State(s) in (\"\")"=w363) -> ("States Out"=w362:string)  [unwired: 14 in]
          }
          frame "---------- Events ----------" {
            # "Template Separator\n(You can make a copy of, or modify, this frame)"
            n131 = call <vilib>:"Add State(s) to Queue__jki_lib_state_machine.vi"("State(s) in (\"\")"=w368) -> ("States Out"=w367:string)  [unwired: 14 in]
          }
          frame "Events: Register" {
            n132 = Unbundle By Name(w374) -> ("SMO"=w375:refnum<class "Inst.Krohn-Hite-7008.lvclass">)
            n133 = call <vilib>:"GetProtectedEvents.vi"("SMO"=w375) -> ("error out"=w373:errorcluster, "SMO Protected Events"=w378:T24, "SMO out"=w372:refnum<class "Inst.Krohn-Hite-7008.lvclass">)  [unwired: 8 in]
            n134 = call "Inst.KH7008.GetPrivateEvents.vi"("Inst.Krohn-Hite-7008 in"=w372) -> ("error out"=w369:errorcluster, "Inst.Krohn-Hite-7008 Private Events"=w370:cluster{"MessageToProcess":refnum<user-event>})  [unwired: 8 in, 1 out]
            n135 = register-events(w378, w370) -> (reference out=w379:refnum<event-registration>, error out=w376:errorcluster)  [unwired: 2 in]
            n136 = Merge Errors(w376, w369, w373, w371) -> (w377:errorcluster)
            n137 = call <vilib>:"Add State(s) to Queue__jki_lib_state_machine.vi"("State(s) in (\"\")"=w381) -> ("States Out"=w380:string)  [unwired: 14 in]
          }
          frame "Events: Unregister" {
            n138 = Unregister For Events(event registration refnum=w384, error in=w383) -> (error out=w382:errorcluster)
            n139 = call <vilib>:"Clear Errors.vi"("error in (no error)"=w382) -> ()  [unwired: 5 in, 2 out]
            n140 = call <vilib>:"Add State(s) to Queue__jki_lib_state_machine.vi"("State(s) in (\"\")"=w387) -> ("States Out"=w386:string)  [unwired: 14 in]
          }
          frame "---------- Instrument ----------" {
            n141 = Unbundle By Name(w389) -> ("SMO"=w388:refnum<class "Inst.Krohn-Hite-7008.lvclass">)
            n142 = Bundle By Name(cluster=w389, "SMO"=w388) -> (w390:T21)
            n143 = call <vilib>:"Add State(s) to Queue__jki_lib_state_machine.vi"("State(s) in (\"\")"=w394) -> ("States Out"=w393:string)  [unwired: 14 in]
          }
          frame "Instrument: Open Hardware" {
            n144 = Unbundle By Name(w399) -> ("SMO"=w398:refnum<class "Inst.Krohn-Hite-7008.lvclass">)
            n145 = call-dynamic "Open Hardware.vi"("error in (no error)"=w397, "Inst.Krohn-Hite-7008 in"=w398) -> ("error out"=w395:errorcluster, "Inst.Krohn-Hite-7008 out"=w396:refnum<class "Inst.Krohn-Hite-7008.lvclass">)  [unwired: 8 in]
            n146 = Bundle By Name(cluster=w399, "SMO"=w396) -> (w400:T21)
            n147 = call <vilib>:"Add State(s) to Queue__jki_lib_state_machine.vi"("State(s) in (\"\")"=w403) -> ("States Out"=w402:string)  [unwired: 14 in]
          }
          frame "Instrument: Get SR" {
            w409 = Inst.KH7008.ProtectedCommands--Enum."setSR" ("Commands")
            # "broadcast to listeners (UI)"
            n148 = Unbundle By Name(w414) -> ("SMO"=w411:refnum<class "Inst.Krohn-Hite-7008.lvclass">)
            n149 = Unbundle By Name(w411) -> ("VISA resource"=w413:refnum<visa-resource-name>)
            n150 = call "Get Installed SR Type.vi"("error in (no error)"=w412, "VISA Refnum in"=w413) -> ("error out"=w410:errorcluster, "SR"=w406:string)  [unwired: 7 in, 1 out]
            n151 = call "Inst.KH7008.MessageFromProcess.vi"("error in (no error)"=w410, "Data"=w406, "Commands"=w409, "Inst.Krohn-Hite-7008 in"=w411) -> ("error out"=w405:errorcluster, "Inst.Krohn-Hite-7008 out"=w408:refnum<class "Inst.Krohn-Hite-7008.lvclass">)  [unwired: 6 in]
            n152 = call-poly <userlib>:"Instrument.sendMessageToProcess.vi"("error in (no error)"=w405, "Data"=w406, "Command"=w409, "Instrument"=w408) -> ("error out"=w404:errorcluster, "Instrument out"=w407:refnum<class "Inst.Krohn-Hite-7008.lvclass">)  [unwired: 6 in]
            n153 = Bundle By Name(cluster=w414, "SMO"=w407) -> (w415:T21)
            n154 = call <vilib>:"Add State(s) to Queue__jki_lib_state_machine.vi"("State(s) in (\"\")"=w418) -> ("States Out"=w417:string)  [unwired: 14 in]
          }
          frame "Instrument: get" {
            n155 = Unbundle By Name(w434) -> ("SMO"=w433:refnum<class "Inst.Krohn-Hite-7008.lvclass">, "MessageToProcess.Message.Command"=w425:string, "MessageToProcess.Message.Data"=w428:variant)
            n156 = call "Inst.KH7008.handleGetCommand.vi"("error in (no error)"=w430, "Data"=w428, "Command in"=w425, "Inst.Krohn-Hite-7008 in"=w433) -> ("error out"=w429:errorcluster, "output cluster"=w423:T15, "Command out"=w427:string, "Inst.Krohn-Hite-7008 out"=w424:refnum<class "Inst.Krohn-Hite-7008.lvclass">)  [unwired: 4 in]
            n157 = Unbundle By Name(w423) -> ("allChannelProperties"=w419:T3)
            n158 = Empty String/Path?(string/path=w427) -> (empty?=w421:bool)
            n159 = Empty Array?(array=w419) -> (empty?=w422:bool)
            n160 = Or(x=w421, y=w422) -> (x .or. y?=w420:bool)
            n161 = case shown="False" w420 {
              tunnel: w424 -> [w447 w453]
              tunnel: [w444 w453] -> w432
              tunnel: [w448 w454] -> w431
              tunnel: w429 -> [w446 w454]
              tunnel: w427 -> [_ _]
              tunnel: [w451 ""] -> w426
              tunnel: w423 -> [w441 _]
              tunnel: w419 -> [w440 _]
              frame False {
                n162 = call <userlib>:"setAllData.vi"("error in (no error)"=w446, "AllData"=w441, "Instrument in"=w447) -> ("error out"=w442:errorcluster, "Instrument out"=w445:refnum<class "Inst.Krohn-Hite-7008.lvclass">)  [unwired: 7 in]
                n163 = call "Inst.KH7008.MessageFromProcess.vi"("error in (no error)"=w442, "Data"=w441, "Commands"=Inst.KH7008.ProtectedCommands--Enum."setAllChannelProperties" ("protectedCommands"), "Inst.Krohn-Hite-7008 in"=w445) -> ("error out"=w439:errorcluster, "Inst.Krohn-Hite-7008 out"=w444:refnum<class "Inst.Krohn-Hite-7008.lvclass">)  [unwired: 6 in]
                n164 = call "Convert_allChannelProperties_to_JSON.vi"("error in (no error)"=w439, "allChannelProperties"=w440) -> ("error out"=w448:errorcluster, "<JSON>"=w450:string)  [unwired: 8 in]
                n165 = Format Into String(format string="Sequence: Status >> \"%s\"", w450) -> (resulting string=w451:string)  [unwired: 2 in, 1 out]
              }
              frame True {
                # "do not send empty data"
              }
            }
            n166 = Bundle By Name(cluster=w434, "SMO"=w432) -> (w435:T21)
            n167 = call <vilib>:"Add State(s) to Queue__jki_lib_state_machine.vi"("State(s) in Front (\"\")"=w426, "State(s) in (\"\")"=w438) -> ("States Out"=w437:string)  [unwired: 13 in]
          }
          frame "Instrument: set" {
            # "confirm settings were saved\n(and also alert UI and other listeners)"
            n168 = Unbundle By Name(w462) -> ("SMO"=w461:refnum<class "Inst.Krohn-Hite-7008.lvclass">, "MessageToProcess.Message.Command"=w457:string, "MessageToProcess.Message.Data"=w456:variant)
            n169 = call "Inst.KH7008.handleSetCommand.vi"("error in (no error)"=w459, "Data"=w456, "Command"=w457, "Inst.Krohn-Hite-7008 in"=w461) -> ("error out"=w458:errorcluster, "Inst.Krohn-Hite-7008 out"=w460:refnum<class "Inst.Krohn-Hite-7008.lvclass">)  [unwired: 6 in]
            n170 = Bundle By Name(cluster=w462, "SMO"=w460) -> (w463:T21)
            n171 = call <vilib>:"Add State(s) to Queue__jki_lib_state_machine.vi"("State(s) in Front (\"\")"="Instrument: get\nInstrument: Log" ("State(s) in Front (\"\")"), "State(s) in (\"\")"=w466) -> ("States Out"=w465:string)  [unwired: 13 in]
          }
          frame "Instrument: Log" {
            n172 = Unbundle By Name(w481) -> ("SMO"=w474:refnum<class "Inst.Krohn-Hite-7008.lvclass">)
            n173 = Unbundle By Name(w474) -> ("model"=w467:string, "device_id"=w468:string, "allChannelProperties"=w469:T3)
            n174 = Get Date/Time In Seconds() -> (seconds since 1Jan1904=w472:timestamp)
            n175 = for {
              tunnel: w469 -> [w492] mode=indexing
              tunnel: w468 -> [w490]
              tunnel: w473 -> [w489]
              tunnel: [w488] -> w479 mode=indexing
              tunnel: w472 -> [w487]
              tunnel: [w487] -> w471 mode=indexing
              tunnel: w467 -> [w486]
              n176 = call "Convert_ChannelProperty_to_JSON.vi"("error in (no error)"=w489, "channelProperties"=w492) -> ("getChannelResponse"=w491:T14)  [unwired: 8 in, 1 out]
              n177 = Bundle By Name(cluster=w491, "model"=w486, "device_id"=w490) -> (w488:T14)
            }
            n178 = call-dynamic "Get SMO Database Paths.vi"("error in (no error)"=w473, "Inst.Krohn-Hite-7008 in"=w474) -> ("error out"=w477:errorcluster, "Paths"=w476:string, "Inst.Krohn-Hite-7008 out"=w475:refnum<class "Inst.Krohn-Hite-7008.lvclass">)  [unwired: 7 in]
            n179 = call <userlib>:"Instrument.logToDatabaseMultiline.vi"("timestamps"=w471, "error in (no error)"=w477, "Data"=w479, "Paths"=w476, "Instrument"=w475) -> ("error out"=w470:errorcluster, "Instrument out"=w478:refnum<class "Inst.Krohn-Hite-7008.lvclass">)  [unwired: 5 in]
            n180 = Bundle By Name(cluster=w481, "SMO"=w478) -> (w482:T21)
            n181 = call <vilib>:"Add State(s) to Queue__jki_lib_state_machine.vi"("State(s) in Front (\"\")"="" ("State(s) in Front (\"\")"), "State(s) in (\"\")"=w485) -> ("States Out"=w484:string)  [unwired: 13 in]
          }
          frame "Instrument: Close Hardware" {
            n182 = Unbundle By Name(w497) -> ("SMO"=w496:refnum<class "Inst.Krohn-Hite-7008.lvclass">)
            n183 = call-dynamic "Close Hardware.vi"("error in (no error)"=w493, "Inst.Krohn-Hite-7008 in"=w496) -> ("error out"=w494:errorcluster, "Inst.Krohn-Hite-7008 out"=w495:refnum<class "Inst.Krohn-Hite-7008.lvclass">)  [unwired: 8 in]
            n184 = Bundle By Name(cluster=w497, "SMO"=w495) -> (w498:T21)
            n185 = call <vilib>:"Add State(s) to Queue__jki_lib_state_machine.vi"("State(s) in (\"\")"=w501) -> ("States Out"=w500:string)  [unwired: 14 in]
          }
          frame "---------- Sequence ----------" {
            n186 = call <vilib>:"Add State(s) to Queue__jki_lib_state_machine.vi"("State(s) in (\"\")"=w506) -> ("States Out"=w505:string)  [unwired: 14 in]
          }
          frame "Sequence: Status" {
            # "Sequence: Status\n(Use this frame to pass the status to the UI, this VI's UI, etc)"
            n187 = call <vilib>:"Add State(s) to Queue__jki_lib_state_machine.vi"("State(s) in (\"\")"=w512) -> ("States Out"=w511:string)  [unwired: 14 in]
            "Status" <- w507
          }
          frame "Sequence: Wait" {
            # "Sequence: Wait\n(Non-Blocking Wait)"
            # "F = repeat this state. wait\nT = go to next state. don't wait"
            n188 = Unbundle By Name(w521) -> ("Running Step"=w514:i32)
            n189 = call <userlib>:"Wait Logic.vi"("error in (no error)"=w517, "Time"=w515) -> ("error out"=w516:errorcluster, "Status String"=w513:string, "Trigger"=w518:bool)  [unwired: 6 in, 1 out]
            n190 = Increment(x=w514) -> (x+1=w528:i32)
            n191 = Select(t=w528, s=w518, f=w514) -> (s? t:f=w519:i32)
            n192 = Select(t=u32 0, s=w518, f=u32 100 ("milliseconds to wait")) -> (s? t:f=w525:u32)
            n193 = call <userlib>:"Wait (ms)__ogtk.vi"("error in (no error)"=w516, "milliseconds to wait"=w525) -> ("error out"=w523:errorcluster)  [unwired: 8 in, 1 out]
            n194 = Bundle By Name(cluster=w521, "Running Step"=w519) -> (w520:T21)
            n195 = call <vilib>:"Build State String with Arguments__JKI_lib_State_Machine.vi"("Arguments (\"\")"=w513, "State"="Sequence: Status") -> ("State with Arguments"=w522:string)  [unwired: 4 in]
            n196 = call <vilib>:"Add State(s) to Queue__jki_lib_state_machine.vi"("State(s) in Front (\"\")"=w522, "State(s) in (\"\")"=w531) -> ("States Out"=w530:string)  [unwired: 13 in]
          }
        }
      }
    }
    frame Error {
    }
  }
  n197 = call-parent "Process.vi"("error in"=w5, "Instrument"=w4) -> ("error out"=w2:errorcluster, "Instrument out"=→"Inst.Krohn-Hite-7008 out":refnum<class "Inst.Krohn-Hite-7008.lvclass">)  [unwired: 8 in]
  n198 = Merge Errors(w2, w1) -> (→"error out":errorcluster)
